vi "PrimaryInterfaceIsNewDataAvailable.vi"(8 "PrimaryInterface":refnum<k24>, 11 "error in":errorcluster) -> (0 "Data available":bool, 3 "error out":errorcluster)   [LabVIEW 2023, in "UnderAutomation.UniversalRobots.lvlib"]
uses:
  UnderAutomation.UniversalRobots.lvlib
  C:/Users/fg/Documents/UniversalRobots.vi/UnderAutomation.UniversalRobots/lib/UnderAutomation.UniversalRobots.dll
  lib/UnderAutomation.UniversalRobots.dll
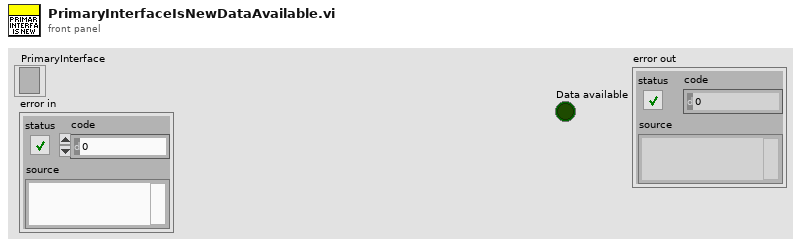
[diagram p1: front panel]
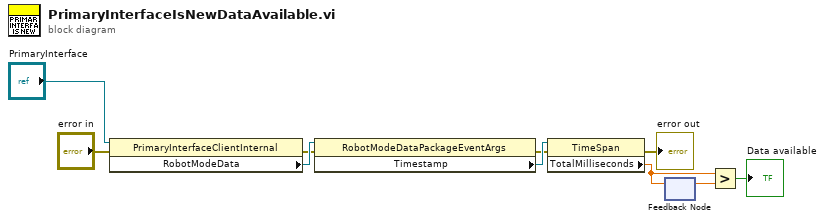
[diagram p0: block diagram]
diagram:
  n1 = property class="PrimaryInterfaceClientInternal"(reference="PrimaryInterface", error in="error in") -> (error out=w3:errorcluster, "RobotModeData"=w10:refnum<k24>)  [unwired: 1 out]
  n2 = property class="RobotModeDataPackageEventArgs"(reference=w10, error in=w3) -> (error out=w2:errorcluster, "Timestamp"=w9:refnum<k24>)  [unwired: 1 out]
  n3 = property class="TimeSpan"(reference=w9, error in=w2) -> (error out=→"error out":errorcluster, "TotalMilliseconds"=w8:dbl)  [unwired: 1 out]
  n4 = feedback #1() -> (w7:dbl)  [unwired: 1 in]
  n5 = feedback-in #1(w8) -> ()
  n6 = Greater?(x=w8, y=w7) -> (0:→"Data available":bool)
